vi "DeQueue ElementsV2.vi"(8 "error in (no error)":errorcluster, 10 "queue in":refnum<queue>, 11 "ChirpV2 in":refnum<class "ChirpV2.lvclass">) -> (0 "error out":errorcluster, 1 "output cluster":T2={"DC_Bias"=0.0, "StartFreq"=0.0, "Duration"=0.0, "State"=enum."Initialization", "window ratio"=0.0, "Final Freq"=0.0}, 2 "queue out":refnum<queue>, 3 "ChirpV2 out":refnum<class "ChirpV2.lvclass">, 5 "#left":i32)   [LabVIEW 2014, in "ChirpV2.lvclass"]
uses:
  ChirpV2.lvclass
  StateV2.ctl
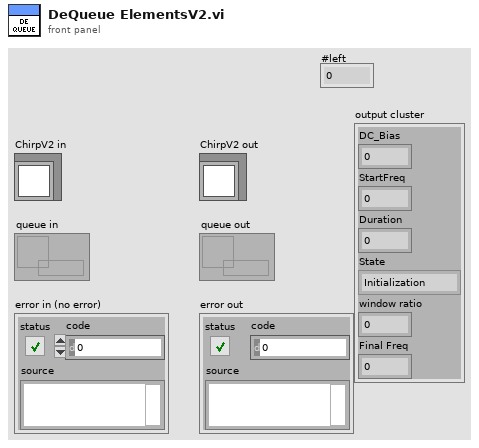
[diagram p1: front panel]
types:
  T1 = typedef "ChirpV2.lvclass/StateV2.ctl" = enum16{"WaitDC", "Initialization", "ChirpSetUp", "Wait", "ChirpMeasurement", "DFT", "WriteData", "Queue", "Ternimation"}
  T2 = cluster{"DC_Bias":dbl, "StartFreq":dbl, "Duration":dbl, "State":T1, "window ratio":dbl, "Final Freq":dbl}
  T3 = cluster{"T":dbl, "Fst":dbl, "Fends":dbl, "Dc":dbl, "w ratio":dbl}
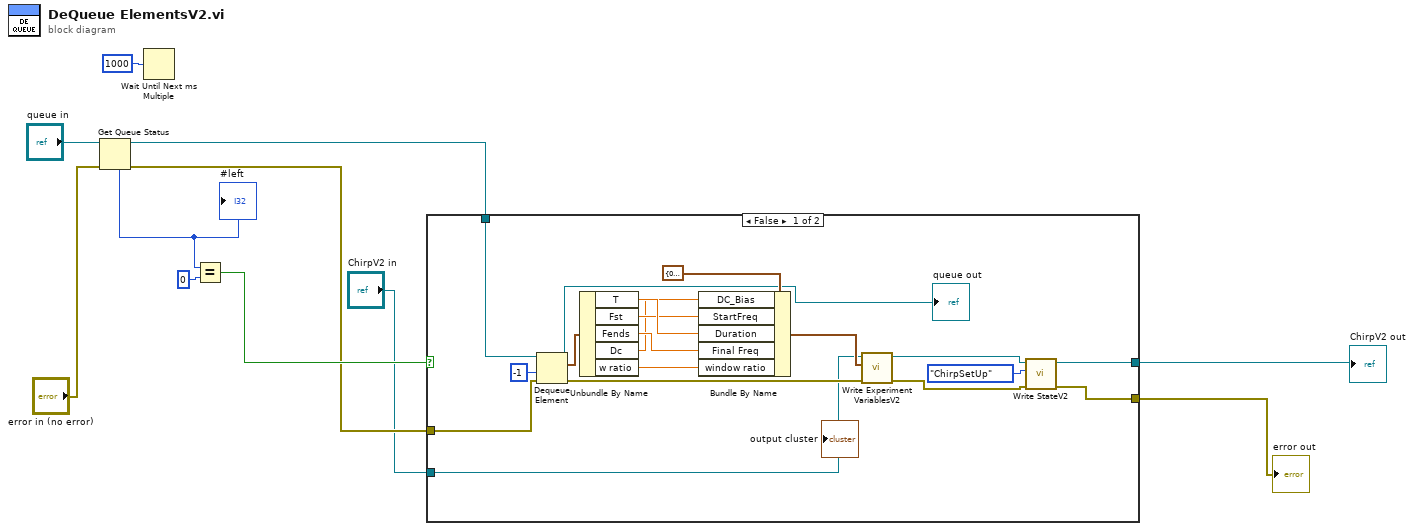
[diagram p0: block diagram]
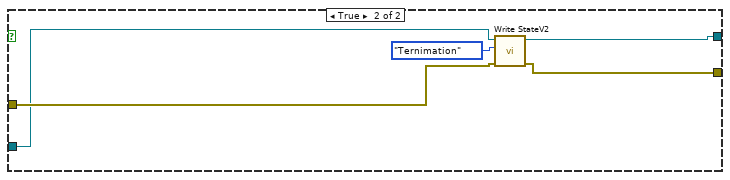
[diagram p2: hidden frame]
diagram:
  n1 = Get Queue Status(queue="queue in", error in (no error)="error in (no error)") -> (queue out=w4:refnum<queue>, error out=w5:errorcluster, # elements in queue=w10:i32)  [unwired: 1 in, 5 out]
  "#left" <- w10
  n2 = Wait Until Next ms Multiple(millisecond multiple=u32 1000) -> ()  [unwired: 1 out]
  n3 = Equal?(x=w10, y=0) -> (x = y?=w7:bool)
  n4 = case shown="False" w7 {
    tunnel: w5 -> [w23 w34]
    tunnel: w4 -> [w22 _]
    tunnel: "ChirpV2 in" -> [w16 w33]
    tunnel: [w15 w32] -> w2
    tunnel: [w14 w31] -> w1
    frame False {
      n5 = Dequeue Element(queue=w22, timeout in ms (-1)=-1, error in (no error)=w23) -> (queue out=→"queue out":refnum<queue>, element=w29:T3, error out=w30:errorcluster)  [unwired: 1 out]
      n6 = Unbundle By Name(w29) -> ("T"=w28:dbl, "Fst"=w27:dbl, "Fends"=w26:dbl, "Dc"=w25:dbl, "w ratio"=w24:dbl)
      n7 = Bundle By Name(cluster=T2 {"DC_Bias"=0.0, "StartFreq"=0.0, "Duration"=0.0, "State"=enum."Initialization", "window ratio"=0.0, "Final Freq"=0.0} ("Experiment Variables"), "DC_Bias"=w25, "StartFreq"=w27, "Duration"=w28, "Final Freq"=w26, "window ratio"=w24) -> (w20:T2)
      n8 = call-dynamic "Write Experiment VariablesV2.vi"("error in (no error)"=w30, "Experiment Variables"=w20, "ChirpV2 in"=w16) -> ("error out"=w17:errorcluster, "ChirpV2 out"=w18:refnum<class "ChirpV2.lvclass">)  [unwired: 7 in]
      n9 = call-dynamic "Write StateV2.vi"("error in (no error)"=w17, "Enum"=StateV2."ChirpSetUp", "ChirpV2 in"=w18) -> ("error out"=w14:errorcluster, "ChirpV2 out"=w15:refnum<class "ChirpV2.lvclass">)  [unwired: 7 in]
    }
    frame True {
      n10 = call-dynamic "Write StateV2.vi"("error in (no error)"=w34, "Enum"=StateV2."Ternimation", "ChirpV2 in"=w33) -> ("error out"=w31:errorcluster, "ChirpV2 out"=w32:refnum<class "ChirpV2.lvclass">)  [unwired: 7 in]
    }
  }
  "ChirpV2 out" <- w2
  "error out" <- w1
